vi "test element.vi"() -> ()   [LabVIEW 2016]
panel:
  out "2D Picture 2":picture
  out "2D Picture":picture
  in  "path to PNG file":path=path "D:/github/Measure_core/Data/settings1_16x16.png"
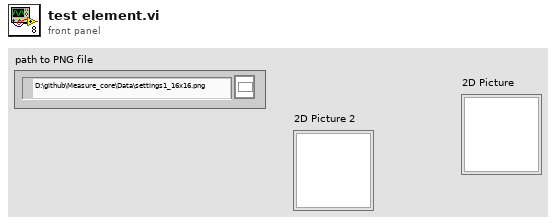
[diagram p1: front panel]
types:
  T1 = typedef "imagedata.ctl" = cluster{"image type":i32, "image depth":i32, "image":u8[], "mask":u8[], "colors":u32[], "Rectangle":cluster{"left":i16, "top":i16, "right":i16, "bottom":i16}}
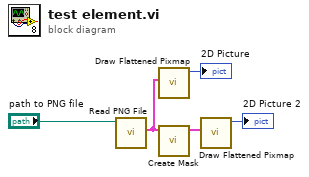
[diagram p0: block diagram]
diagram:
  n1 = call <vilib>:"Read PNG File.vi"("path to PNG file"="path to PNG file") -> ("image data"=w3:T1)  [unwired: 8 in, 2 out]
  n2 = call <vilib>:"Draw Flattened Pixmap.vi"("image data"=w3) -> ("new picture"=→"2D Picture":picture)  [unwired: 8 in]
  n3 = call <vilib>:"Create Mask.vi"("image data"=w3) -> ("image data"=w2:T1)  [unwired: 10 in]
  n4 = call <vilib>:"Draw Flattened Pixmap.vi"("image data"=w2) -> ("new picture"=→"2D Picture 2":picture)  [unwired: 8 in]
